vi "CalculateFPS.vi"(2 "Update interval":u32=1000, 3 "buffer number":u32) -> (0 "processed FPS":dbl, 1 "acquired FPS":dbl)   [LabVIEW 2025]
doc: "Calculate the frame rate from within a loop. Frame rate is averaged over the specified update interval. The default update interval is 1000ms."
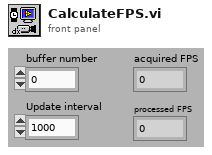
[diagram p1: front panel]
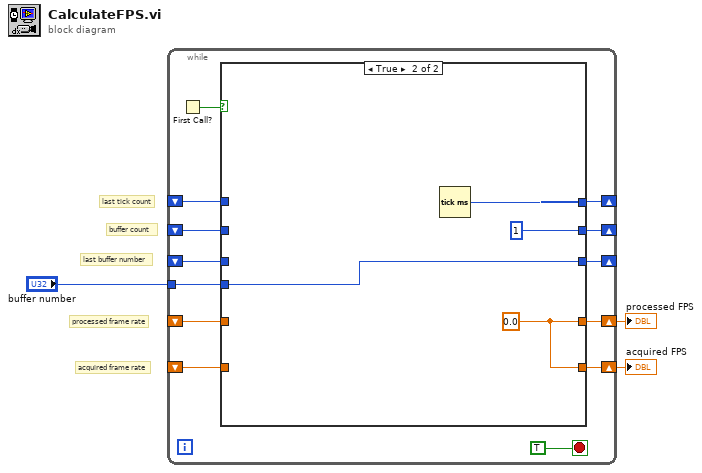
[diagram p0: block diagram]
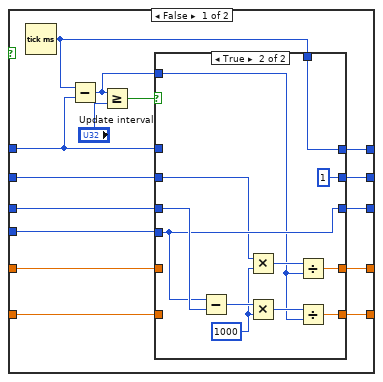
[diagram p2: hidden frame]
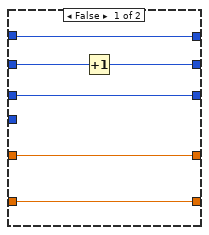
[diagram p3: hidden frame]
diagram:
  # "processed frame rate"
  # "buffer count"
  # "last buffer number"
  # "acquired frame rate"
  # "last tick count"
  n1 = while {
    shift-right: [w14] -> _
    shift-left: _ -> [w13]
    shift-right: [w11] -> _
    shift-left: _ -> [w12]
    shift-right: [w10] -> w3
    shift-left: _ -> [w9]
    tunnel: "buffer number" -> [w8]
    shift-right: [w7] -> _
    shift-left: _ -> [w6]
    shift-right: [w5] -> w1
    shift-left: _ -> [w4]
    stop <- TRUE stop-if-true
    n2 = First Call?() -> (First Call?: T/F=w15:bool)
    n3 = case shown="True" w15 {
      tunnel: [w28 w53] -> w14
      tunnel: w13 -> [w29 _]
      tunnel: w12 -> [w27 _]
      tunnel: [w26 w52] -> w11
      tunnel: [w23 w50] -> w10
      tunnel: w9 -> [w22 _]
      tunnel: w8 -> [w21 w52]
      tunnel: [w19 u32 1 ("buffer number")] -> w7
      tunnel: w6 -> [w20 _]
      tunnel: [w18 w50] -> w5
      tunnel: w4 -> [w17 _]
      frame False {
        n4 = Tick Count (ms)() -> (millisecond timer value=w25:u32)
        n5 = Subtract(x=w25, y=w29) -> (x-y=w24:u32)
        n6 = Greater Or Equal?(x=w24, y="Update interval") -> (x >= y?=w30:bool)
        n7 = case shown="True" w30 {
          tunnel: w29 -> [w37 _]
          tunnel: [w37 w49] -> w28
          tunnel: w27 -> [w35 w45]
          tunnel: [w35 w44] -> w26
          tunnel: w25 -> [_ w49]
          tunnel: w24 -> [_ w39]
          tunnel: [w36 w47] -> w23
          tunnel: w22 -> [w36 _]
          tunnel: w21 -> [_ w44]
          tunnel: w20 -> [w34 w41]
          tunnel: [w33 u32 1] -> w19
          tunnel: [w32 w38] -> w18
          tunnel: w17 -> [w32 _]
          frame False {
            n8 = Increment(x=w34) -> (x+1=w33:u32)
          }
          frame True {
            w42 = u32 1000 ("y")
            n9 = Subtract(x=w44, y=w45) -> (x-y=w46:u32)
            n10 = Multiply(x=w41, y=w42) -> (x*y=w40:u32)
            n11 = Multiply(x=w46, y=w42) -> (x*y=w48:u32)
            n12 = Divide(x=w40, y=w39) -> (x/y=w38:dbl)
            n13 = Divide(x=w48, y=w39) -> (x/y=w47:dbl)
          }
        }
      }
      frame True {
        w50 = 0.0
        n14 = Tick Count (ms)() -> (millisecond timer value=w53:u32)
      }
    }
  }
  "acquired FPS" <- w3
  "processed FPS" <- w1
